vi "Autonomous State Machine Straight.vi"() -> ()   [LabVIEW 2014]
doc: "This VI is called when autonomous begins, and will automatically be terminated when autonomous ends. You can carry out timed or sensor driven robot movement independently without needing to return to the caller."
uses:
  <vilib>/Rock Robotics/WPI/RobotDrive/WPI_RobotDriveGetSetRefNum.vi
panel:
  in  "power":dbl=-0.7 format="%#_13g"
  # "Be sure to right-click and choose Data Operations>>Make Current Value default if you want to save the array values with the VI"
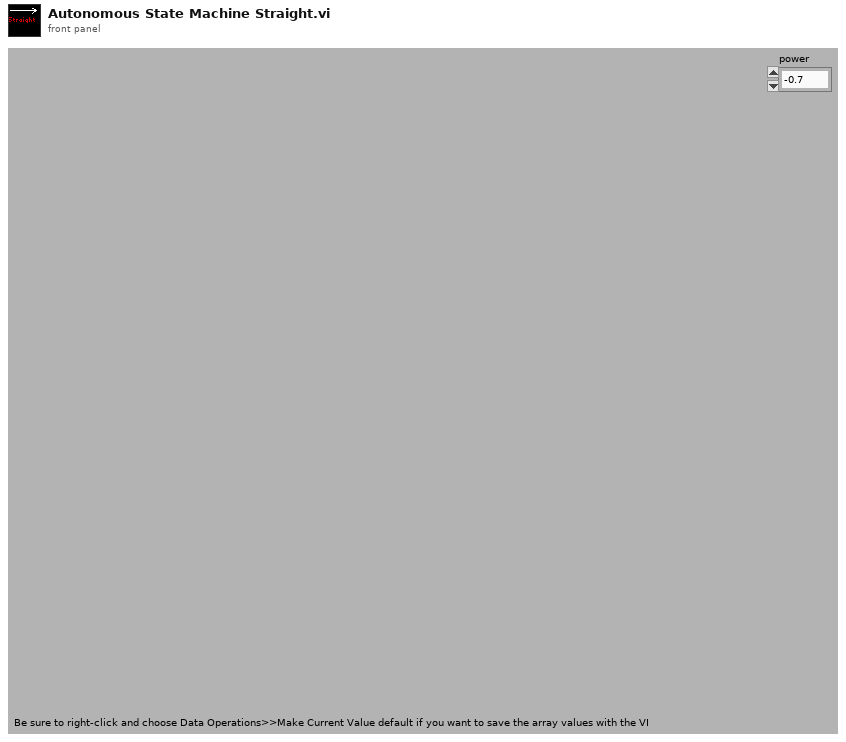
[diagram p1: front panel]
types:
  T1 = typedef "WPI_EncoderDevRef.ctl" = cluster{"DevStatus":errorcluster, "EncoderIndex":T2, "CounterIndex":T3, "DistancePerCount":dbl, "Decoding Type":T4}
  T2 = typedef "FPGA_EncoderIdx.ctl" = enum8{"Enc 0", "Enc 1", "Enc 2", "Enc 3", "Enc 4", "Enc 5", "Enc 6", "Enc 7", "Invalid"}
  T3 = typedef "FPGA_CounterCtrSystemIndex.ctl" = enum8{"Ctr 0", "Ctr 1", "Ctr 2", "Ctr 3", "Ctr 4", "Ctr 5", "Ctr 6", "Ctr 7", "Invalid"}
  T4 = typedef "WPI_EncoderType.ctl" = enum16{"1x", "2x", "4x"}
  T5 = typedef "WPI_RobotDriveDevRef.ctl" = cluster{"DevStatus":errorcluster, "Motors[]":T6[], "Square Inputs":bool, "Max Output":dbl}
  T6 = typedef "WPI_MotorControlDeviceRef.ctl" = cluster{"DeviceStatus":errorcluster, "Type":T7, "PWM":cluster{"Controller":T8, "PWM Channel":T9, "DeadBand":T10}, "CAN":cluster{"Device Number":u8, "Control Mode":T11, "Semaphore":T12, "Max Vout":dbl, "TalonSRX Control Mode":T13}, "Invert":bool, "TransformRef":T14, "InvTransformRef":T14}
  T7 = typedef "WPI_MotorControlType.ctl" = enum16{"PWM", "CAN", "CANTalonSRX"}
  T8 = typedef "FPGA_TypedefDigitalModule.ctl" = enum16{"Controller 1"}
  T9 = typedef "FPGA_DIOPWMChannel.ctl" = enum8{"PWM 0", "PWM 1", "PWM 2", "PWM 3", "PWM 4", "PWM 5", "PWM 6", "PWM 7", "PWM 8", "PWM 9", "PWM MXP 0", "PWM MXP 1", "PWM MXP 2", "PWM MXP 3", "PWM MXP 4", "PWM MXP 5", "PWM MXP 6", "PWM MXP 7", "PWM MXP 8", "PWM MXP 9", "Invalid"}
  T10 = typedef "WPI_PWMDeadband.ctl" = cluster{"Name":string, "maxPositivePwm":i32, "minPositivePwm":i32, "centerPwm":i32, "maxNegativePwm":i32, "minNegativePwm":i32, "angularRange":u16}
  T11 = typedef "WPI_CANJaguar_ControlMode.ctl" = enum8{"Percent VBus", "Current", "Speed", "Position", "Voltage"}
  T12 = typedef "Semaphore RefNum" = refnum<k1>
  T13 = typedef "WPI_CANTalonSRX_APIControlMode.ctl" = enum8{"Percent VBus", "Speed", "Position", "Slave", "Unchanged / Invalid"}
  T14 = typedef "WPI_PWMTransform_ConPane.ctl" = refnum<vi>
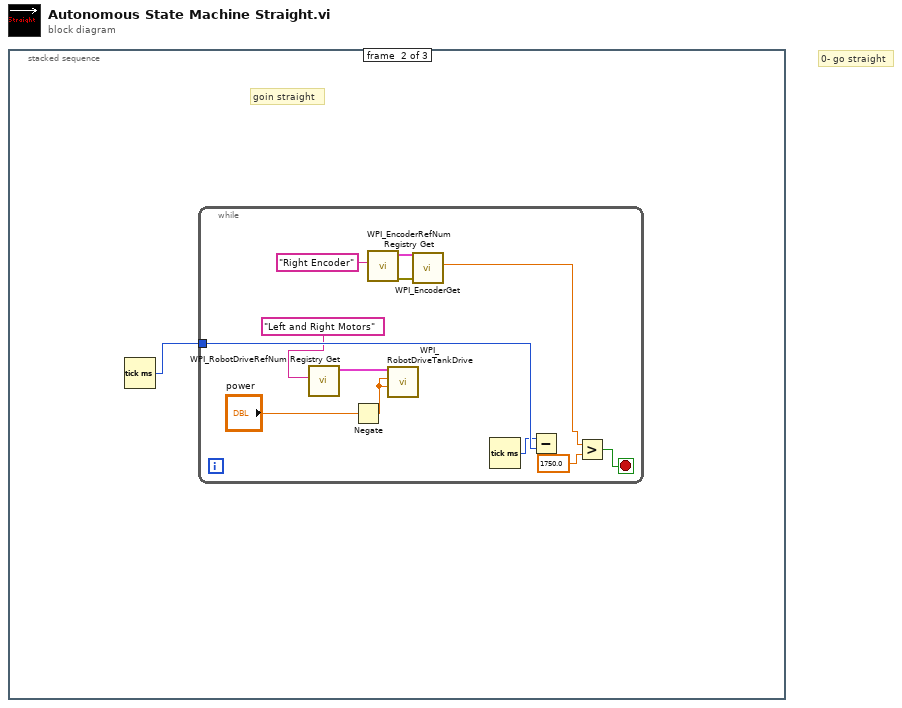
[diagram p0: block diagram]
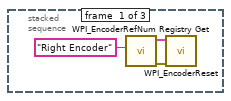
[diagram p2: hidden frame]
diagram:
  # "0- go straight"
  n1 = stacked-sequence {
    frame #0 {
      n2 = call <vilib>:"WPI_EncoderRefNum Registry Get.vi"("refnum name"="Right Encoder") -> ("error out"=w2:errorcluster, "EncoderDevRef"=w1:T1)  [unwired: 9 in]
      n3 = call <vilib>:"WPI_EncoderReset.vi"("error in (no error)"=w2, "EncoderDevRef"=w1) -> ()  [unwired: 8 in, 2 out]
    }
    frame #1 {
      # "goin straight"
      n4 = Tick Count (ms)() -> (millisecond timer value=w4:u32)
      n5 = while {
        tunnel: w4 -> [w15]
        stop <- w16 stop-if-true
        n6 = call <vilib>:"WPI_RobotDriveRefNum Registry Get.vi"("refnum name"="Left and Right Motors") -> ("RobotDriveDevRef"=w13:T5)  [unwired: 9 in, 1 out]
        n7 = Negate(x="power") -> (-x=w5:dbl)
        n8 = call <vilib>:"WPI_EncoderRefNum Registry Get.vi"("refnum name"="Right Encoder") -> ("error out"=w9:errorcluster, "EncoderDevRef"=w8:T1)  [unwired: 9 in]
        n9 = call <vilib>:"WPI_RobotDriveTankDrive.vi"("Right axis value"=w5, "Left axis value"=w5, "RobotDriveDevRef"=w13) -> ()  [unwired: 6 in, 3 out]
        n10 = call <vilib>:"WPI_EncoderGet.vi"("error in (no error)"=w9, "EncoderDevRef"=w8) -> ("Distance"=w7:dbl)  [unwired: 4 in, 5 out]
        n11 = Tick Count (ms)() -> (millisecond timer value=w14:u32)
        n12 = Subtract(x=w14, y=w15) -> ()  [unwired: 1 out]
        n13 = Greater?(x=w7, y=1750.0 ("x")) -> (0:w16:bool)
      }
    }
    frame #2 {
    }
  }
